vi "Close.vi"(8 "error in (no error)":errorcluster, 11 "NI Switch in":refnum<class "NI Switch.lvclass">) -> (0 "error out":errorcluster, 3 "NI Switch out":refnum<class "NI Switch.lvclass">)   [LabVIEW 2025, in "Switch.lvlib" / "NI Switch.lvclass"]
uses:
  NI Switch.lvclass
  NI Switch.lvclass/NI Switch.ctl
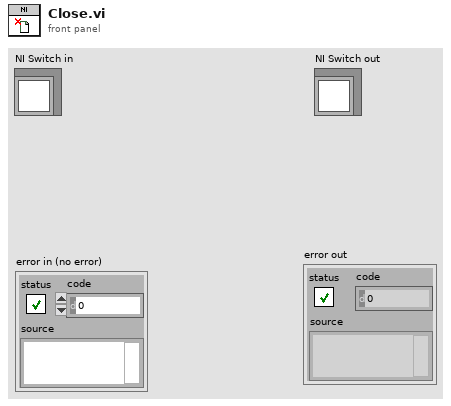
[diagram p1: front panel]
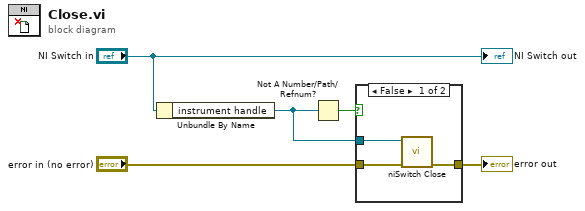
[diagram p0: block diagram]
diagram:
  n1 = Unbundle By Name("NI Switch in") -> ("instrument handle"=w1:refnum<k15>)
  n2 = Not A Number/Path/Refnum?(number/path/refnum=w1) -> (NaN/Path/Refnum?=w2:bool)
  n3 = case shown="False" w2 {
    tunnel: "error in (no error)" -> [w8 w9]
    tunnel: [w7 w9] -> w3
    tunnel: w1 -> [w6 _]
    frame False {
      n4 = call <instrlib>:"niSwitch Close.vi"("error in (no error)"=w8, "instrument handle"=w6) -> ("error out"=w7:errorcluster)  [unwired: 9 in]
    }
    frame True {
    }
  }
  "error out" <- w3
  "NI Switch out" <- "NI Switch in"
